vi "Build AND List.vi"(11 "String Array":string[](array[string])) -> (3 "AND String":string)   [LabVIEW 2011]
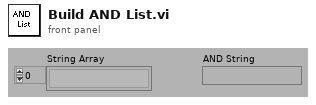
[diagram p1: front panel]
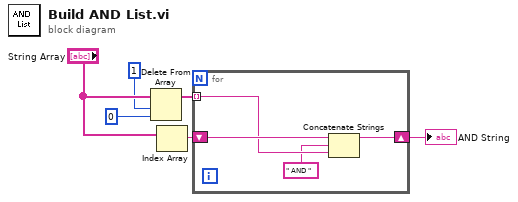
[diagram p0: block diagram]
diagram:
  n1 = Delete From Array(array="String Array", length=1 ("y"), index=0 ("y")) -> (array with subset deleted=w4:string[])  [unwired: 1 out]
  n2 = Index Array(array="String Array") -> (element=w2:string)  [unwired: 1 in]
  n3 = for {
    shift-right: [w7] -> w6
    shift-left: w2 -> [w10]
    tunnel: w4 -> [w9] mode=indexing
    n4 = Concatenate Strings(w10, " AND ", w9) -> (w7:string)
  }
  "AND String" <- w6
